vi "Pre Launch Init.vi"(11 "Nested in":refnum<class "Msg.lvclass">) -> (0 "error out":errorcluster, 3 "Nested out":refnum<class "Msg.lvclass">)   [LabVIEW 2020, in "Msg.lvlib" / "Msg.lvclass"]
doc: "(<B>Filename</B>: Actor Framework.lvlib:Actor.lvclass:Pre Launch Init.vi)\n\nDefines behavior that occurs after the Launch Nested Actor method is invoked but before the actor's Actor Core method begins running.\n\nBy default, this method does nothing. A descendant class may override it to define behavior."
uses:
  Msg.lvclass
  C:/Program Files (x86)/National Instruments/LabVIEW 2020/vi.lib/ActorFramework/Actor/Actor.lvclass
  Msg.lvclass/Msg.ctl
  <vilib>/ActorFramework/Actor/Actor.lvclass/Actor.ctl
  <vilib>/ActorFramework/Message Enqueuer/Message Enqueuer.lvclass/Message Enqueuer.ctl
  <vilib>/ActorFramework/Message Enqueuer/Init from Existing Queue.vi
  <vilib>/ActorFramework/Message Enqueuer/Enqueue.vi
  Msg Messages/Init Msg/Init Msg.lvclass
  C:/Program Files (x86)/National Instruments/LabVIEW 2020/vi.lib/ActorFramework/Message/Message.lvclass
  <vilib>/ActorFramework/Message Priority Queue/Priority Enqueue.vi
  <vilib>/ActorFramework/Message Enqueuer/Message Enqueuer.lvclass
  <vilib>/ActorFramework/Actor/Actor.lvclass
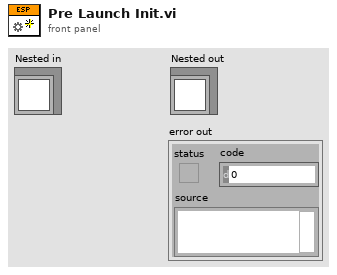
[diagram p1: front panel]
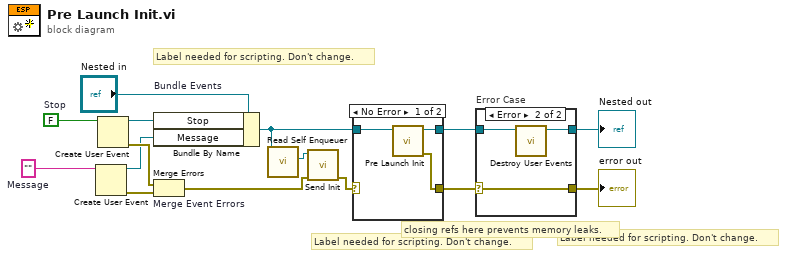
[diagram p0: block diagram]
diagram:
  w7 = ""  # Message
  w14 = FALSE  # Stop
  # "Label needed for scripting. Don't change."
  # "Label needed for scripting. Don't change."
  # "Label needed for scripting. Don't change."
  # "closing refs here prevents memory leaks."
  n1 = Create User Event(user event datatype=w7) -> (user event=w6:refnum<user-event>, error out=w5:errorcluster)  [unwired: 1 in]
  n2 = Create User Event(user event datatype=w14) -> (user event=w11:refnum<user-event>, error out=w13:errorcluster)  [unwired: 1 in]
  n3 = Bundle By Name "Bundle Events"(cluster="Nested in", "Stop"=w11, "Message"=w6) -> (w4:refnum<class "Msg.lvclass">)
  n4 = Merge Errors "Merge Event Errors"(w13, w5) -> (w2:errorcluster)
  n5 = call <vilib>:"Read Self Enqueuer.vi"("Actor"=w4) -> ("Self Enqueuer"=w3:refnum<class "Message Enqueuer.lvclass">)  [unwired: 10 in]
  n6 = call "Send Init.vi"("error in (no error)"=w2, "Message Enqueuer"=w3) -> ("error out"=w1:errorcluster)  [unwired: 8 in, 1 out]
  n7 = case shown="No Error" w1 {
    selector: w1 -> [_ w20]
    tunnel: [w18 w19] -> w9
    tunnel: w4 -> [w17 w19]
    tunnel: [w16 w20] -> w8
    frame No Error {
      n8 = call-parent "Pre Launch Init.vi"("Actor in"=w17) -> ("error out"=w16:errorcluster, "Actor out"=w18:refnum<class "Msg.lvclass">)  [unwired: 9 in]
    }
    frame Error {
    }
  }
  n9 = case "Error Case" shown="Error" w8 {
    selector: w8 -> [w21 w25]
    tunnel: w9 -> [w22 w24]
    tunnel: [w22 w23] -> w12
    tunnel: [w21 w25] -> w10
    frame No Error {
    }
    frame Error {
      n10 = call "Destroy User Events.vi"("UI Template in"=w24) -> ("UI Template out"=w23:refnum<class "Msg.lvclass">)  [unwired: 10 in]
    }
  }
  "error out" <- w10
  "Nested out" <- w12
